vi "Tools_Windows Open Regional Settings Dialog.vi"(8 "error in (no error)":errorcluster, 10 "Wait until dialog is closed":bool=TRUE) -> (0 "error out":errorcluster)   [LabVIEW 2014]
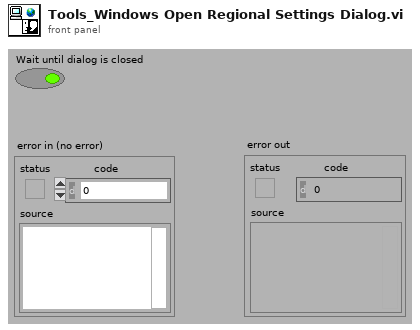
[diagram p1: front panel]
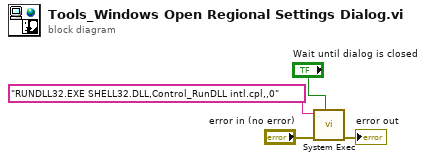
[diagram p0: block diagram]
diagram:
  n1 = call <vilib>:"System Exec.vi"("wait until completion? (T)"="Wait until dialog is closed", "error in (no error)"="error in (no error)", "command line"="RUNDLL32.EXE SHELL32.DLL,Control_RunDLL intl.cpl,,0") -> ("error out"=→"error out":errorcluster)  [unwired: 5 in, 3 out]
